vi "QueuedStateMachine-Ext.vi"() -> ()   [LabVIEW 2020]
panel:
  out "DataRx":i32
  in  "TxData":T1
  out "error out":errorcluster
  in  "error in":errorcluster
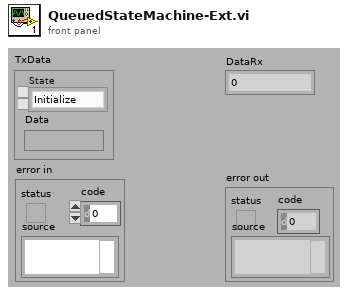
[diagram p1: front panel]
types:
  T1 = cluster{"Data":variant, "State":enum16{"Initialize", "TX", "RX", "STOP"}}
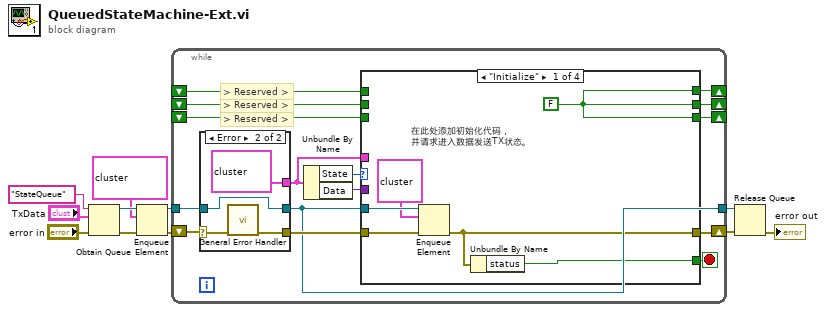
[diagram p0: block diagram]
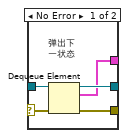
[diagram p2: hidden frame]
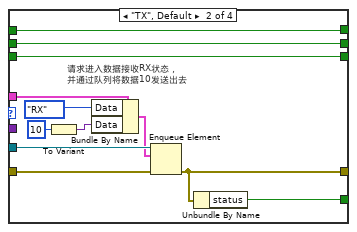
[diagram p3: hidden frame]
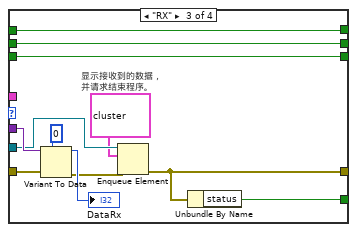
[diagram p4: hidden frame]
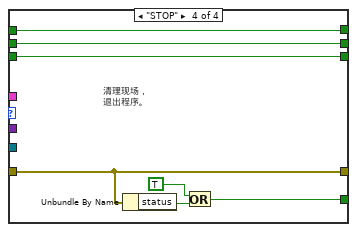
[diagram p5: hidden frame]
diagram:
  n1 = Obtain Queue(name (unnamed)="StateQueue", element data type="TxData", error in (no error)="error in") -> (queue out=w10:refnum<queue>, error out=w9:errorcluster)  [unwired: 2 in, 1 out]
  n2 = Enqueue Element(queue=w10, element=T1 {"Data"=variant, "State"=enum."Initialize"} ("Queue Data"), error in (no error)=w9) -> (queue out=w3:refnum<queue>, error out=w2:errorcluster)  [unwired: 1 in, 1 out]
  n3 = while {
    shift-right: [w25] -> w8
    shift-left: w2 -> [w17]
    shift-right: [w21] -> _
    shift-left: _ -> [w19]
    shift-right: [w24] -> _
    shift-left: _ -> [w22]
    shift-right: [w23] -> _
    shift-left: _ -> [w20]
    tunnel: w3 -> [w18]
    tunnel: [w15] -> w7
    stop <- w26 stop-if-true
    # "> Reserved >"
    # "> Reserved >"
    # "> Reserved >"
    n4 = case shown="Error" w17 {
      selector: w17 -> [w30 w35]
      tunnel: w18 -> [w31 w34]
      tunnel: [w29 w34] -> w15
      tunnel: [w28 w33] -> w16
      tunnel: [w27 T1 {"Data"=variant, "State"=enum."STOP"} ("Queue Data")] -> w12
      frame No Error {
        # "弹出下\n一状态"
        n5 = Dequeue Element(queue=w31, error in (no error)=w30) -> (queue out=w29:refnum<queue>, element=w27:T1, error out=w28:errorcluster)  [unwired: 1 in, 1 out]
      }
      frame Error {
        n6 = call <vilib>:"General Error Handler.vi"("error in (no error)"=w35) -> ("error out"=w33:errorcluster)  [unwired: 10 in, 4 out]
      }
    }
    n7 = Unbundle By Name(w12) -> ("State"=w14:enum16{"Initialize", "TX", "RX", "STOP"}, "Data"=w13:variant)
    n8 = case shown="\"Initialize\"" w14 {
      tunnel: [w40 w50 w62 w68] -> w26
      tunnel: w16 -> [w39 w53 w60 w69]
      tunnel: [w38 w51 w54 w69] -> w25
      tunnel: [w41 w48 w64 w71] -> w24
      tunnel: [w41 w47 w65 w70] -> w23
      tunnel: w22 -> [_ w48 w64 w71]
      tunnel: [w41 w49 w63 w72] -> w21
      tunnel: w20 -> [_ w47 w65 w70]
      tunnel: w19 -> [_ w49 w63 w72]
      tunnel: w15 -> [w37 w52 w56 _]
      tunnel: w13 -> [_ _ w61 _]
      tunnel: w12 -> [_ w46 _ _]
      frame "Initialize" {
        w41 = FALSE
        # "在此处添加初始化代码，\n并请求进入数据发送TX状态。"
        n9 = Enqueue Element(queue=w37, element=T1 {"Data"=variant, "State"=enum."TX"} ("Queue Data"), error in (no error)=w39) -> (error out=w38:errorcluster)  [unwired: 1 in, 2 out]
        n10 = Unbundle By Name(w38) -> ("status"=w40:bool)
      }
      frame "TX", Default {
        # "请求进入数据接收RX状态，\n并通过队列将数据10发送出去"
        n11 = To Variant(anything=10) -> (Variant=w43:variant)
        n12 = Bundle By Name(cluster=w46, "Data"=enum16{"Initialize", "TX", "RX", "STOP"}."RX" ("State"), "Data"=w43) -> (w45:T1)
        n13 = Enqueue Element(queue=w52, element=w45, error in (no error)=w53) -> (error out=w51:errorcluster)  [unwired: 1 in, 2 out]
        n14 = Unbundle By Name(w51) -> ("status"=w50:bool)
      }
      frame "RX" {
        # "显示接收到的数据，\n并请求结束程序。"
        n15 = Variant To Data(error in=w60, type=0, Variant=w61) -> (data=→"DataRx":i32, error out=w57:errorcluster)
        n16 = Enqueue Element(queue=w56, element=T1 {"Data"=variant, "State"=enum."STOP"} ("Queue Data"), error in (no error)=w57) -> (error out=w54:errorcluster)  [unwired: 1 in, 2 out]
        n17 = Unbundle By Name(w54) -> ("status"=w62:bool)
      }
      frame "STOP" {
        # "清理现场，\n退出程序。"
        n18 = Unbundle By Name(w69) -> ("status"=w67:bool)
        n19 = Or(x=TRUE, y=w67) -> (x .or. y?=w68:bool)
      }
    }
  }
  n20 = Release Queue(queue=w7, error in (no error)=w8) -> (error out=→"error out":errorcluster)  [unwired: 1 in, 2 out]
